vi "Elevator Tuner.vi"() -> ()   [LabVIEW 2018]
uses:
  TrapezoidalMotionProfile/Constraints.ctl
  TrapezoidalMotionProfile/TrapezoidalProfile.lvclass
  <vilib>/Rock Robotics/WPI/ThirdParty/REV Robotics/SPARK MAX/Typedef/Spark MAX Control Type.ctl
  TrapezoidalMotionProfile/State.ctl
panel:
  out "Motor Temperature":u8=48
  out "current (A)":dbl
  out "Current":dbl=0.125
  out "Applied Output":dbl=-0.0
  out "Sensor Position":dbl
  out "TrapezoidalProfile out":refnum<class "TrapezoidalProfile.lvclass">
  in  "Radio Buttons":T1(radio)=enum."Motion Profile"
  in  "Slide":dbl(slide)=0.06122448979591821 scale=-1.0..1.0
  in  "Max Velocity (RPS)":dbl=10.0 format="%#_13g"
  in  "PID Constants":T2={"P Gain"=0.5, "I Gain"=0.0, "D Gain"=0.0, "F Gain"=0.0, "I Zone"=0.0, "Min Output"=-1.0, "Max Output"=1.0}
  in  "Setpoint":dbl
  out "Waveform Chart":T3(graph)={"Position (u)"=0.0, "Sensor Position"=0.0, "Velocity (u/s)"=0.0, "Sensor Velocity"=-0.0}
  in  "Elevator Constraints":T4={"Max Velocity"=40.0, "Max Accel"=50.0}
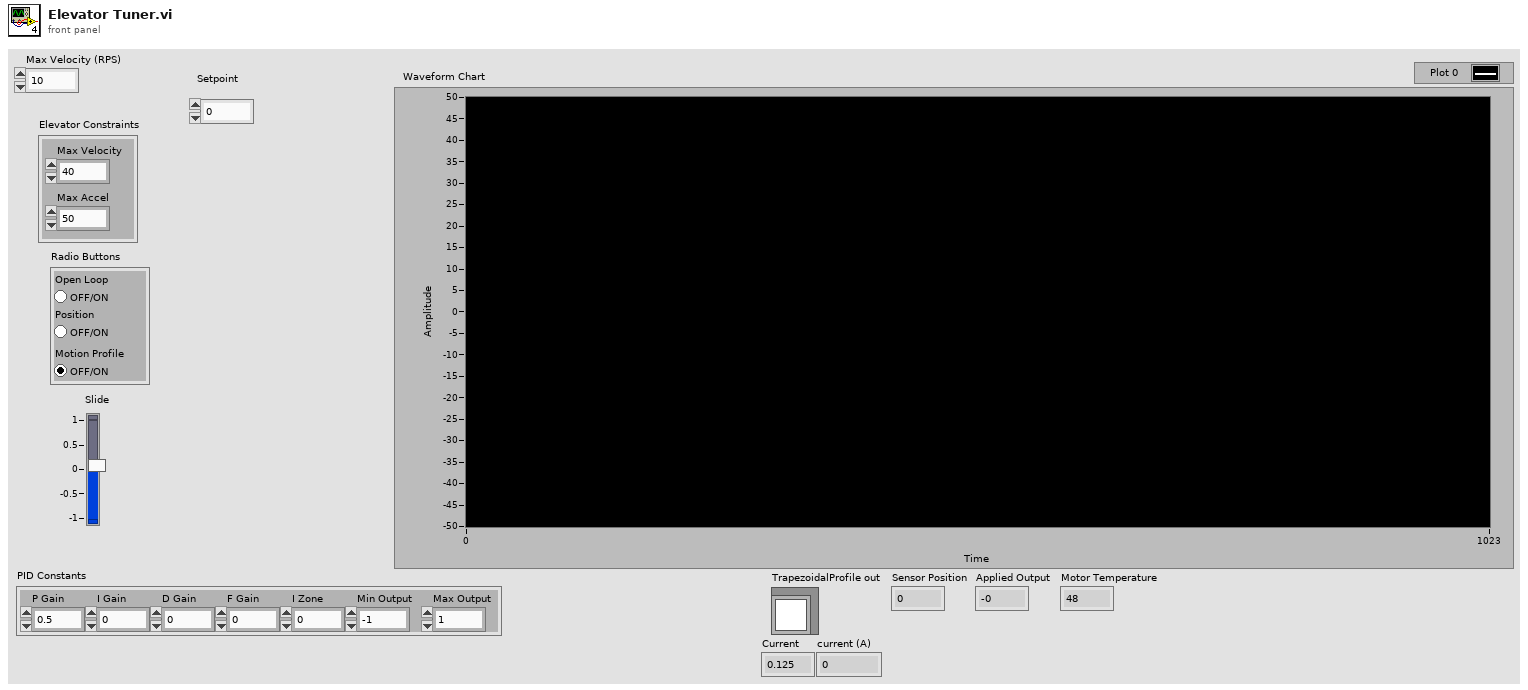
[diagram p1: front panel]
types:
  T1 = enum32{"Open Loop", "Position", "Motion Profile"}
  T2 = cluster{"P Gain":dbl, "I Gain":dbl, "D Gain":dbl, "F Gain":dbl, "I Zone":dbl, "Min Output":dbl, "Max Output":dbl}
  T3 = cluster{"Position (u)":dbl, "Sensor Position":dbl, "Velocity (u/s)":dbl, "Sensor Velocity":dbl}
  T4 = typedef "TrapezoidalProfile.lvclass/Constraints.ctl" = cluster{"Max Velocity":dbl, "Max Accel":dbl}
  T5 = typedef "WPI_MotorControlDeviceRef.ctl" = cluster{"DeviceStatus":errorcluster, "Type":T6, "PWM":cluster{"PWM Channel":T7, "DeadBand":T8}, "CAN":cluster{"Device Number":u8, "SetOutput VI Ref":variant, "GetOutput VI Ref":variant, "Enable VI Ref":variant, "Disable VI Ref":variant, "Data":variant}, "Invert":bool, "DIO PWM":cluster{"PWM \"Enable\" Channel":T7, "DIOChannel":T9, "PWM Rate":dbl}}
  T6 = typedef "WPI_MotorControlType.ctl" = enum16{"PWM", "CAN", "DIO PWM"}
  T7 = typedef "FPGA_DIOPWMChannel.ctl" = enum8{"PWM 0", "PWM 1", "PWM 2", "PWM 3", "PWM 4", "PWM 5", "PWM 6", "PWM 7", "PWM 8", "PWM 9", "PWM MXP 0", "PWM MXP 1", "PWM MXP 2", "PWM MXP 3", "PWM MXP 4", "PWM MXP 5", "PWM MXP 6", "PWM MXP 7", "PWM MXP 8", "PWM MXP 9", "Invalid"}
  T8 = typedef "WPI_PWMDeadband.ctl" = cluster{"Name":string, "maxPositivePwm":i32, "minPositivePwm":i32, "centerPwm":i32, "maxNegativePwm":i32, "minNegativePwm":i32, "angularRange":u16}
  T9 = typedef "FPGA_DIOChannel.ctl" = enum8{"DIO 0", "DIO 1", "DIO 2", "DIO 3", "DIO 4", "DIO 5", "DIO 6", "DIO 7", "DIO 8", "DIO 9", "DIO MXP 0", "DIO MXP 1", "DIO MXP 2", "DIO MXP 3", "DIO MXP 4", "DIO MXP 5", "DIO MXP 6", "DIO MXP 7", "DIO MXP 8", "DIO MXP 9", "DIO MXP 10", "DIO MXP 11", "DIO MXP 12", "DIO MXP 13", "DIO MXP 14", "DIO MXP 15", "SPI Port CS1", "SPI Port CS2", "SPI Port CS3", "SPI Port MISO", "SPI Port MOSI", "Invalid"}
  T10 = cluster{"P Gain":bool, "I Gain":bool, "D Gain":bool, "F Gain":bool, "I Zone":bool, "Min Output":bool, "Max Output":bool}
  T11 = typedef "TrapezoidalProfile.lvclass/State.ctl" = cluster{"Position (u)":dbl, "Velocity (u/s)":dbl}
  T12 = typedef "Spark MAX Control Type.ctl" = enum16{"Percent VBus", "Voltage", "Velocity", "Position", "Smart Motion", "Current", "Smart Velocity"}
  T13 = cluster{"Setpoint":dbl, "Sensor Position":dbl, "Velocity (u/s)":dbl, dbl}
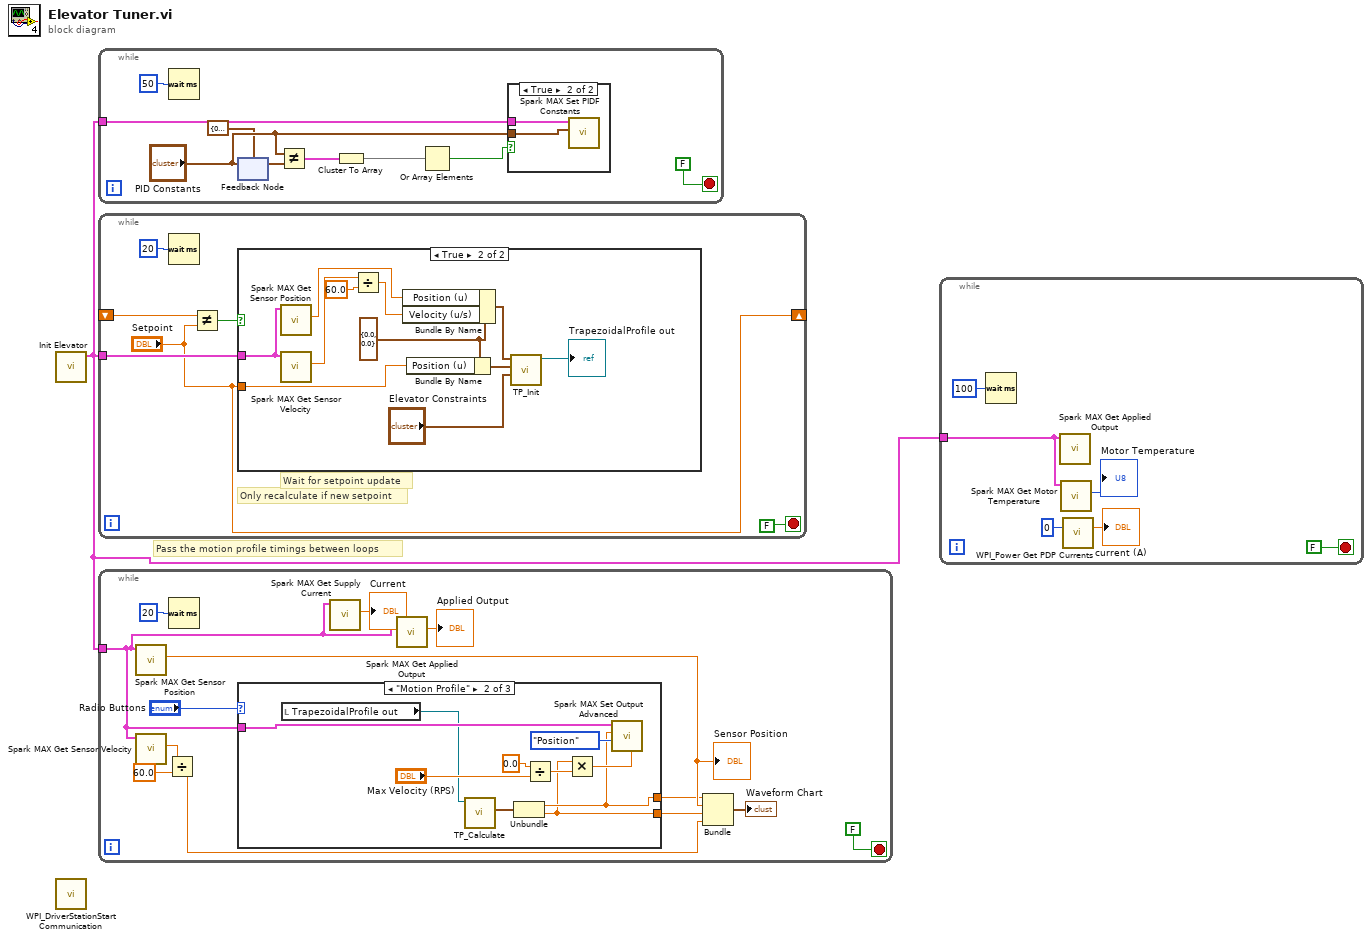
[diagram p0: block diagram]
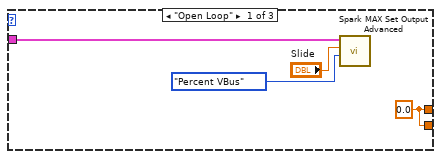
[diagram p3: hidden frame]
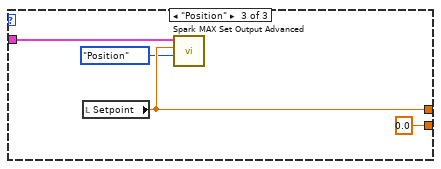
[diagram p4: hidden frame]
diagram:
  # "Pass the motion profile timings between loops"
  n1 = call "Init Elevator.vi"() -> ("Master Out"=w1:T5)  [unwired: 10 in, 1 out]
  n2 = call <vilib>:"WPI_DriverStationStart Communication.vi"() -> ()  [unwired: 12 in]
  n3 = while {
    tunnel: w1 -> [w6]
    stop <- FALSE stop-if-true
    n4 = Wait (ms)(milliseconds to wait=u32 50) -> ()  [unwired: 1 out]
    n5 = feedback-in #1("PID Constants") -> ()
    n6 = feedback #1(T2 {"P Gain"=0.0, "I Gain"=0.0, "D Gain"=0.0, "F Gain"=0.0, "I Zone"=0.0, "Min Output"=0.0, "Max Output"=0.0} ("PID Constants")) -> (w10:T2)
    n7 = Not Equal?(x="PID Constants", y=w10) -> (x != y?=w9:T10)
    n8 = Cluster To Array(cluster=w9) -> (array=w8:bool[])
    n9 = Or Array Elements(Boolean array=w8) -> (logical OR=w7:bool)
    n10 = case shown="True" w7 {
      tunnel: w6 -> [_ w12]
      tunnel: "PID Constants" -> [_ w11]
      frame False {
      }
      frame True {
        n11 = call <vilib>:"Spark MAX Set PIDF Constants.vi"("PID Constants"=w11, "MotorControlDeviceRef"=w12) -> ()  [unwired: 8 in, 2 out]
      }
    }
  }
  n12 = while {
    shift-right: ["Setpoint"] -> _
    shift-left: _ -> [w16]
    tunnel: w1 -> [w15]
    stop <- FALSE stop-if-true
    # "Only recalculate if new setpoint"
    # "Wait for setpoint update"
    n13 = Wait (ms)(milliseconds to wait=u32 20) -> ()  [unwired: 1 out]
    n14 = Not Equal?(x=w16, y="Setpoint") -> (x != y?=w18:bool)
    n15 = case shown="True" w18 {
      tunnel: "Setpoint" -> [_ w28]
      tunnel: w15 -> [_ w25]
      frame False {
      }
      frame True {
        w19 = T11 {"Position (u)"=0.0, "Velocity (u/s)"=0.0} ("Unprofiled Goal")
        n16 = call <vilib>:"Spark MAX Get Sensor Position.vi"("MotorControlDevRef in"=w25) -> ("Sensor Position"=w24:dbl)  [unwired: 7 in, 3 out]
        n17 = call <vilib>:"Spark MAX Get Sensor Velocity.vi"("MotorControlDevRef in"=w25) -> ("Sensor Velocity"=w22:dbl)  [unwired: 7 in, 3 out]
        n18 = Divide(x=w22, y=60.0) -> (x/y=w21:dbl)
        n19 = Bundle By Name(cluster=w19, "Position (u)"=w24, "Velocity (u/s)"=w21) -> (w20:T11)
        n20 = Bundle By Name(cluster=w19, "Position (u)"=w28) -> (w27:T11)
        n21 = call "TP_Init.vi"("Constraints"="Elevator Constraints", "Unprofiled Goal"=w27, "Initial"=w20) -> ("TrapezoidalProfile out"=→"TrapezoidalProfile out":refnum<class "TrapezoidalProfile.lvclass">)  [unwired: 7 in, 1 out]
      }
    }
  }
  n22 = while {
    tunnel: w1 -> [w31]
    stop <- FALSE stop-if-true
    n23 = call <vilib>:"Spark MAX Get Sensor Position.vi"("MotorControlDevRef in"=w31) -> ("Sensor Position"=w40:dbl)  [unwired: 7 in, 3 out]
    "Sensor Position" <- w40
    n24 = call <vilib>:"Spark MAX Get Sensor Velocity.vi"("MotorControlDevRef in"=w31) -> ("Sensor Velocity"=w39:dbl)  [unwired: 7 in, 3 out]
    n25 = Divide(x=w39, y=60.0) -> (x/y=w34:dbl)
    n26 = Wait (ms)(milliseconds to wait=u32 20) -> ()  [unwired: 1 out]
    n27 = case shown="\"Motion Profile\"" "Radio Buttons" {
      tunnel: w31 -> [w46 w55 w60]
      tunnel: [w45 w49 w59] -> w38
      tunnel: [w45 w48 0.0 ("Velocity (u/s)")] -> w37
      frame "Open Loop" {
        w45 = 0.0 ("Setpoint")
        n28 = call <vilib>:"Spark MAX Set Output Advanced.vi"("Control Mode"=Spark_MAX_Control_Type."Percent VBus", "Setpoint"="Slide", "MotorControlDevRef"=w46) -> ()  [unwired: 7 in, 2 out]
      }
      frame "Motion Profile" {
        n29 = local read "TrapezoidalProfile out"() -> (w47:refnum<class "TrapezoidalProfile.lvclass">)
        n30 = call "TP_Calculate.vi"("TrapezoidalProfile in"=w47) -> ("Output"=w51:T11)  [unwired: 8 in, 2 out]
        n31 = Unbundle(w51) -> ("Position (u)"=w49:dbl, "Velocity (u/s)"=w48:dbl)
        n32 = Divide(x=0.0, y="Max Velocity (RPS)") -> (x/y=w54:dbl)
        n33 = Multiply(x=w48, y=w54) -> (x*y=w50:dbl)
        n34 = call <vilib>:"Spark MAX Set Output Advanced.vi"("Arbitrary Feed Forward (0)"=w50, "Control Mode"=Spark_MAX_Control_Type."Position", "Setpoint"=w49, "MotorControlDevRef"=w55) -> ()  [unwired: 6 in, 2 out]
      }
      frame "Position" {
        n35 = local read "Setpoint"() -> (w59:dbl)
        n36 = call <vilib>:"Spark MAX Set Output Advanced.vi"("Control Mode"=Spark_MAX_Control_Type."Position", "Setpoint"=w59, "MotorControlDevRef"=w60) -> ()  [unwired: 7 in, 2 out]
      }
    }
    n37 = call <vilib>:"Spark MAX Get Supply Current.vi"("MotorControlDevRef in"=w31) -> ("Current"=→"Current":dbl)  [unwired: 7 in, 3 out]
    n38 = call <vilib>:"Spark MAX Get Applied Output.vi"("MotorControlDevRef in"=w31) -> ("Applied Output"=→"Applied Output":dbl)  [unwired: 7 in, 3 out]
    n39 = Bundle("Setpoint"=w38, "Sensor Position"=w40, "Velocity (u/s)"=w37, w34) -> (→"Waveform Chart":T13)  [unwired: 1 in]
  }
  n40 = while {
    tunnel: w1 -> [w63]
    stop <- FALSE stop-if-true
    n41 = Wait (ms)(milliseconds to wait=u32 100) -> ()  [unwired: 1 out]
    n42 = call <vilib>:"Spark MAX Get Applied Output.vi"("MotorControlDevRef in"=w63) -> ()  [unwired: 7 in, 4 out]
    n43 = call <vilib>:"Spark MAX Get Motor Temperature.vi"("MotorControlDevRef in"=w63) -> ("Motor Temperature"=→"Motor Temperature":u8)  [unwired: 7 in, 3 out]
    n44 = call <vilib>:"WPI_Power Get PDP Currents.vi"("PDP Channel"=0) -> ("current (A)"=→"current (A)":dbl)  [unwired: 12 in, 2 out]
  }
